vi "Open Deployable Packed Library.vi"(8 "error in (no error)":errorcluster, 10 "Build specification name":string, 11 "TargetItem Refnum":refnum<vi>) -> (0 "error out":errorcluster, 3 "PPL out":refnum<class "NI_AB_API_DPPL.lvclass">)   [LabVIEW 2020, in "NI_AB_API_DPPL.lvclass"]
uses:
  <vilib>/AppBuilder/AB_API/DPPL/NI_AB_API_DPPL.lvclass
  e:/builds/penguin/labview/branches/2020/dev/dist/vi.lib/AppBuilder/AB_API/Build/NI_AB_API_Build.lvclass
  <vilib>/AppBuilder/AB_API/common/AB_API Build Object Type.ctl
  <vilib>/AppBuilder/AB_Classes/Build/AB_Build.lvclass
  <vilib>/AppBuilder/AB_API/Build/NI_AB_API_Build.lvclass
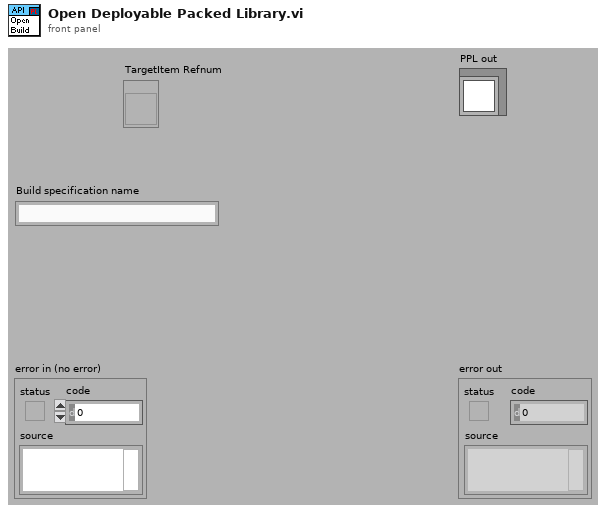
[diagram p1: front panel]
types:
  T1 = typedef "AB_API Build Object Type.ctl" = enum16{"Source Distribution", "DLL", "EXE", "Installer", "Zip File", "RESTful WS", "RTEXE", "Packed Library", "C Generation ", ".NET Interop Assembly"}
  T2 = typedef "ItemRef.ctl" = u64
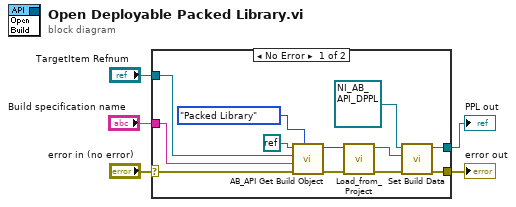
[diagram p0: block diagram]
diagram:
  n1 = case shown="No Error" "error in (no error)" {
    selector: "error in (no error)" -> [w12 w18]
    tunnel: [w9 w18] -> w4
    tunnel: [w7 _] -> w3
    tunnel: "TargetItem Refnum" -> [w14 _]
    tunnel: "Build specification name" -> [w13 _]
    frame No Error {
      n2 = call <vilib>:"AB_API Get Build Object.vi"("Build object type"=AB_API_Build_Object_Type."Packed Library", "error in (no error)"=w12, "Build spec name"=w13, "TargetItem Refnum"=w14, "Project Refnum"=refnum<k0> refnum) -> ("error out"=w15:errorcluster, "Build Object"=w16:T2)  [unwired: 5 in]
      n3 = call <vilib>:"Load_from_Project.vi"("error in (no error)"=w15, "Object"=w16) -> ("error out"=w10:errorcluster, "Build out"=w6:refnum<class "AB_Build.lvclass">)  [unwired: 8 in]
      n4 = call <vilib>:"Set Build Data.vi"("error in (no error)"=w10, "AB_Build.lvclass"=w6, "NI_AB_API_Build in"=refnum<class "NI_AB_API_DPPL.lvclass"> refnum ("NI_AB_API_DLL.lvclass")) -> ("error out"=w9:errorcluster, "NI_AB_API_Build out"=w7:refnum<class "NI_AB_API_DPPL.lvclass">)  [unwired: 7 in]
    }
    frame Error {
    }
  }
  "error out" <- w4
  "PPL out" <- w3
